vi "temperature.vi"() -> ()   [LabVIEW 2021]
uses:
  <vilib>/addons/control/pid/pid.llb/PID (DBL).vi
  <vilib>/addons/control/pid/NI_PID_pid.lvlib
panel:
  out "设定温度与当前温度差":dbl
  out "当前温度":dbl(slide) scale=0.0..100.0
  in  "PID gains":T1={"proportional gain (Kc)"=1.0, "integral time (Ti, min)"=0.01, "derivative time (Td, min)"=0.0} caption="PID增益" {"derivative time (Td, min)" format="%.3f"; "integral time (Ti, min)" format="%.3f"; "proportional gain (Kc)" format="%.3f"}
  in  "设定温度":dbl(knob) min=0.0 max=50.0 step=1.0 scale=0.0..50.0
  out "温度控制波形图":cluster{"设备输出":dbl, "设定温度":dbl}(graph)
  in  "停止":bool
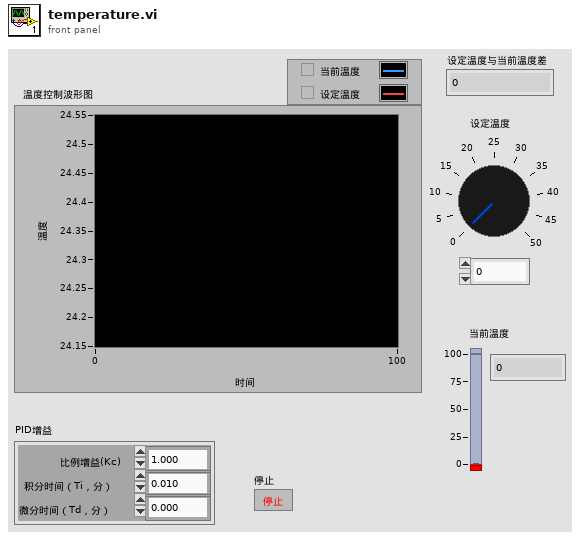
[diagram p1: front panel]
types:
  T1 = cluster{"proportional gain (Kc)":dbl, "integral time (Ti, min)":dbl, "derivative time (Td, min)":dbl}
  T2 = cluster{"static gain":dbl, "lag (min)":dbl, "dead cycles":dbl, "load %":dbl, "deadband":dbl, "noise level %":dbl, "initial PV":dbl, "initial PV 2":dbl}
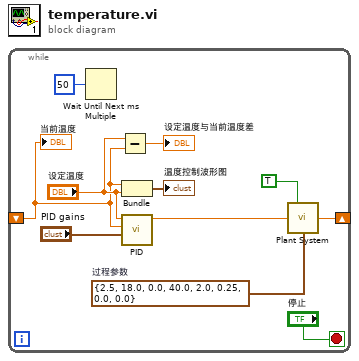
[diagram p0: block diagram]
diagram:
  n1 = while {
    shift-right: [w8] -> _
    shift-left: _ -> [w2]
    stop <- "停止" stop-if-true
    w4 = T2 {"static gain"=2.5, "lag (min)"=18.0, "dead cycles"=0.0, "load %"=40.0, "deadband"=2.0, "noise level %"=0.25, "initial PV"=0.0, "initial PV 2"=0.0}  # 过程参数
    n2 = Wait Until Next ms Multiple(millisecond multiple=u32 50 ("毫秒计时值")) -> ()  [unwired: 1 out]
    n3 = Subtract(x="设定温度", y=w2) -> (x-y=→"设定温度与当前温度差":dbl)
    n4 = Bundle("设备输出"=w2, "设定温度"="设定温度") -> (→"温度控制波形图":cluster{"设备输出":dbl, "设定温度":dbl})  [unwired: 1 in]
    n5 = call-poly <vilib>:"PID.vi"("PID gains"="PID gains", "process variable"=w2, "setpoint"="设定温度") -> ("output"=w9:dbl)  [unwired: 7 in, 1 out]
    n6 = call "Plant System.vi"("积分器？"=TRUE ("Integrator ?"), "设备输入"=w9, "过程参数"=w4) -> ("设备输出"=w8:dbl)  [unwired: 12 in]
    "当前温度" <- w2
  }
